vi "ReadBounds.vi"(8 "error in (no error)":errorcluster) -> (0 "error out":errorcluster, 3 "Bounds":T1)   [LabVIEW 2017, in "DisplayWindow.lvlib" / "DisplayWindow.lvclass"]
doc: "Read the boundaries of the DisplayWindow from the configuration file."
uses:
  DisplayWindow.lvclass
  <vilib>/Utility/miscctls.llb/LVRectTypeDef.ctl
  <vilib>/Utility/config.llb/Read Key (I32).vi
  <vilib>/Utility/config.llb/NI_LVConfig.lvlib
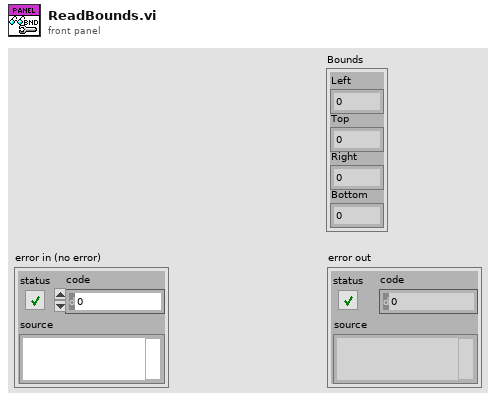
[diagram p1: front panel]
types:
  T1 = typedef "LVRectTypeDef.ctl" = cluster{"Left":i16, "Top":i16, "Right":i16, "Bottom":i16}
  T2 = typedef "NI_LVConfig.lvlib/Config Data RefNum.ctl" = refnum<k1>
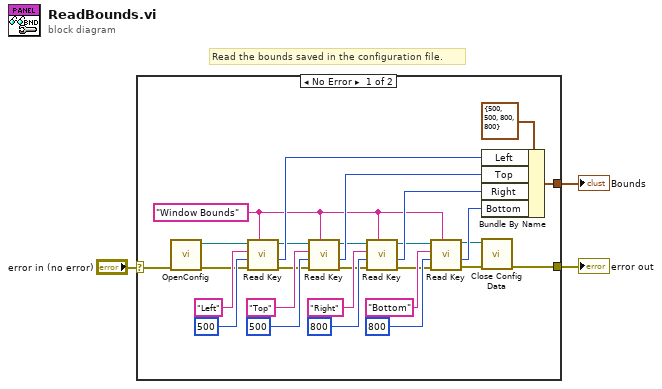
[diagram p0: block diagram]
diagram:
  # "Read the bounds saved in the configuration file."
  n1 = case shown="No Error" "error in (no error)" {
    selector: "error in (no error)" -> [w26 w31]
    tunnel: [w25 w31] -> w2
    tunnel: [w8 _] -> w1
    frame No Error {
      w18 = "Window Bounds"
      n2 = call "OpenConfig.vi"("error in (no error)"=w26) -> ("error out"=w7:errorcluster, "refnum"=w24:T2)  [unwired: 9 in]
      n3 = call-poly <vilib>:"Read Key.vi"("section"=w18, "error in (no error)"=w7, "default value"=500, "key"="Left", "refnum"=w24) -> ("error out"=w6:errorcluster, "value"=w29:i32, "refnum out"=w23:T2)  [unwired: 3 in, 1 out]
      n4 = call-poly <vilib>:"Read Key.vi"("section"=w18, "error in (no error)"=w6, "default value"=500, "key"="Top", "refnum"=w23) -> ("error out"=w5:errorcluster, "value"=w30:i32, "refnum out"=w22:T2)  [unwired: 3 in, 1 out]
      n5 = call-poly <vilib>:"Read Key.vi"("section"=w18, "error in (no error)"=w5, "default value"=800, "key"="Right", "refnum"=w22) -> ("error out"=w4:errorcluster, "value"=w27:i32, "refnum out"=w21:T2)  [unwired: 3 in, 1 out]
      n6 = call-poly <vilib>:"Read Key.vi"("section"=w18, "error in (no error)"=w4, "default value"=800, "key"="Bottom", "refnum"=w21) -> ("error out"=w19:errorcluster, "value"=w28:i32, "refnum out"=w20:T2)  [unwired: 3 in, 1 out]
      n7 = Bundle By Name(cluster=T1 {"Left"=500, "Top"=500, "Right"=800, "Bottom"=800} ("Bounds"), "Left"=w29, "Top"=w30, "Right"=w27, "Bottom"=w28) -> (w8:T1)
      n8 = call <vilib>:"Close Config Data.vi"("error in (no error)"=w19, "refnum"=w20) -> ("error out"=w25:errorcluster)  [unwired: 8 in, 1 out]
    }
    frame Error {
    }
  }
  "error out" <- w2
  "Bounds" <- w1
